vi "Vision Processing.vi"(4 "error in (no error)":errorcluster) -> ()   [LabVIEW 2015]
doc: "This VI runs in parallel to other tasks. It gets images from the camera, processes them for color or shape and use that information to affect robot behavior."
uses:
  <vilib>/Rock Robotics/SystemInterfaces/NetworkCommunication/NetComm_UsageReport_ResourceType.ctl
  <vilib>/Rock Robotics/WPI/Camera/WPI_CameraExposure Values.ctl
  <vilib>/Rock Robotics/WPI/Utilities/WPI_GetSetVariantRefNum.vi
  <vilib>/Rock Robotics/Network Tables/NT Write Boolean.vi
  Robot Global Data.vi
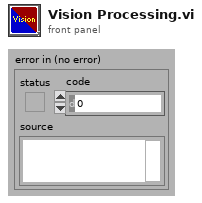
[diagram p1: front panel]
types:
  T1 = typedef "WPI_CameraExposure Values.ctl" = enum16{"Auto", "Flicker-free 50 Hz", "Flicker-free 60 Hz", "Hold current", "Custom"}
  T2 = cluster{"fps":i32, "compression":i32, "compression 2":i32}
  T3 = typedef "NetComm_UsageReport_ResourceType.ctl" = enum8{"Controller", "Module", "Language", "CANPlugin", "Accelerometer", "ADXL345", "AnalogChannel", "AnalogTrigger", "AnalogTriggerOutput", "CANJaguar", "Compressor", "Counter", "Dashboard", "DigitalInput", "DigitalOutput", "DriverStationCIO", "DriverStationEIO", "DriverStationLCD", "Encoder", "GearTooth", "Gyro", "I2C", "Framework", "Jaguar", "Joystick", "Kinect", "KinectStick", "PIDController", "Preferences", "PWM", "Relay", "RobotDrive", "SerialPort", "Servo", "Solenoid", "SPI", "Task", "Ultrasonic", "Victor", "Button", "Command", "AxisCamera", "PCVideoServer", "SmartDashboard", "Talon", "HiTechnicColorSensor", "HiTechnicAccel", "HiTechnicCompass", "SRF08", "AnalogOutput", "Victor SP", "Talon SRX", "CAN Talon SRX", "ADXL362 Accel", "ADXRS450 Gyro", "Rev SPARK", "Mindsensors SD540", "Digital Filter"}
  T4 = enum16{"Update Mode", "Get Image", "Get Image Data"}
  T5 = typedef "WPI_JoystickDevRef.ctl" = cluster{"Device":T6}
  T6 = typedef "WPI_JoystickDeviceEnum.ctl" = enum16{"USB 0", "USB 1", "USB 2", "USB 3", "USB 4", "USB 5"}
  T7 = typedef "WPI_CameraDevRef.ctl" = cluster{"Camera Address":string, "CameraStatus":errorcluster}
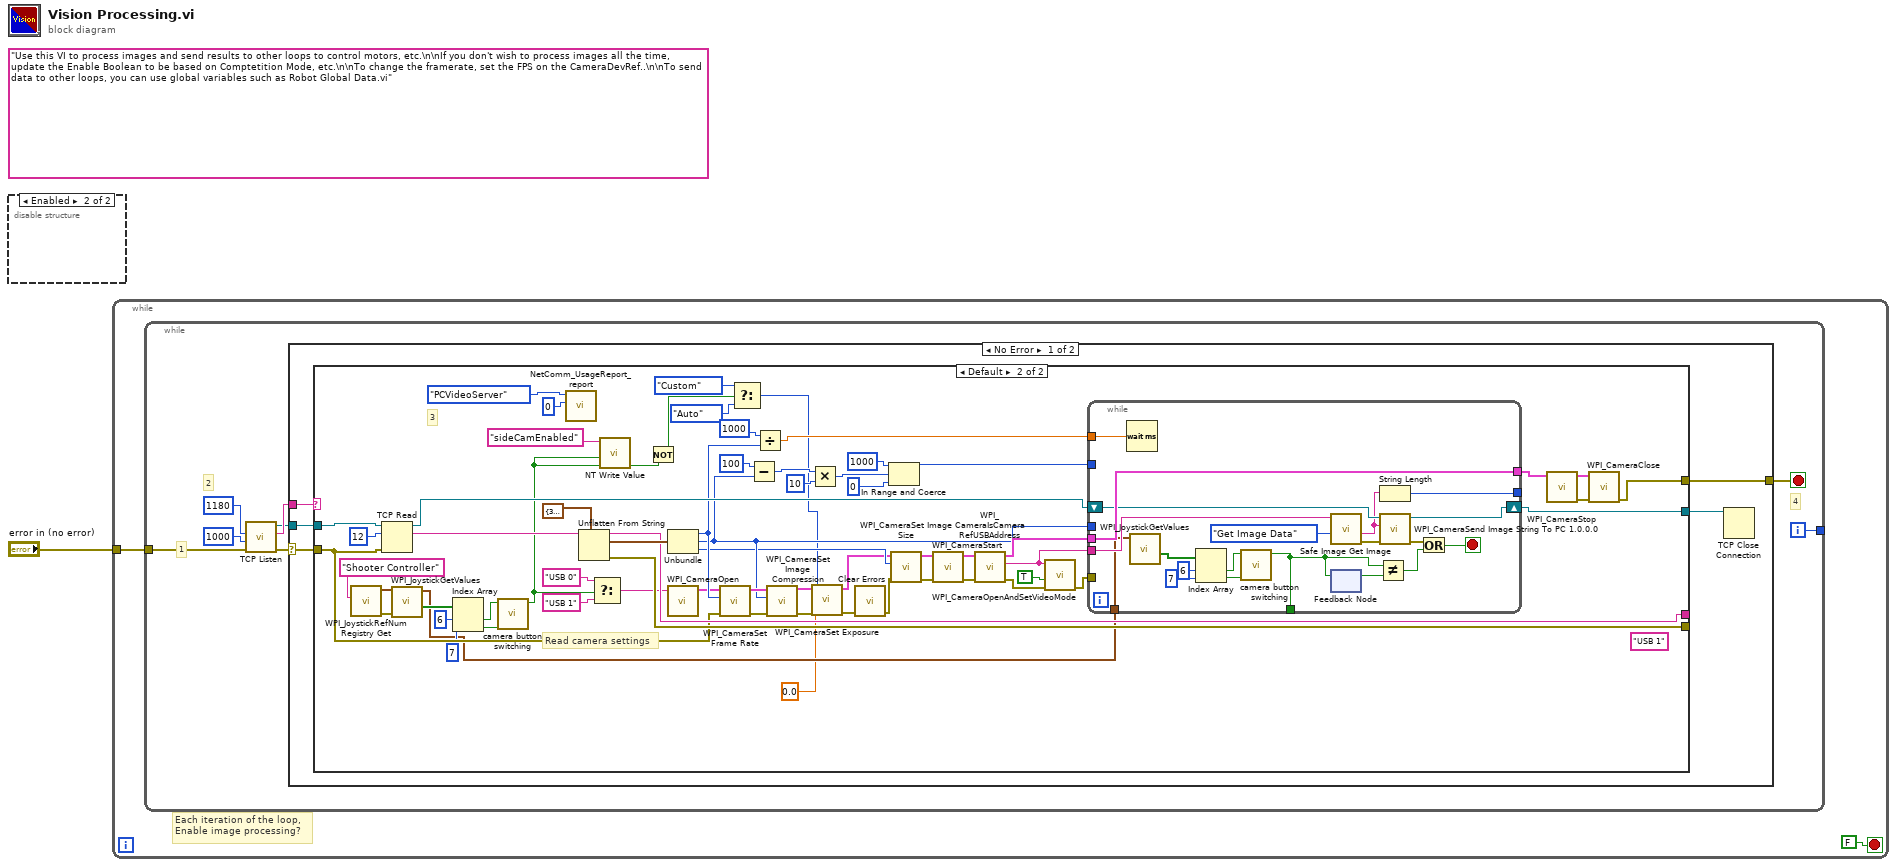
[diagram p0: block diagram]
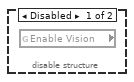
[diagram p2: hidden frame]
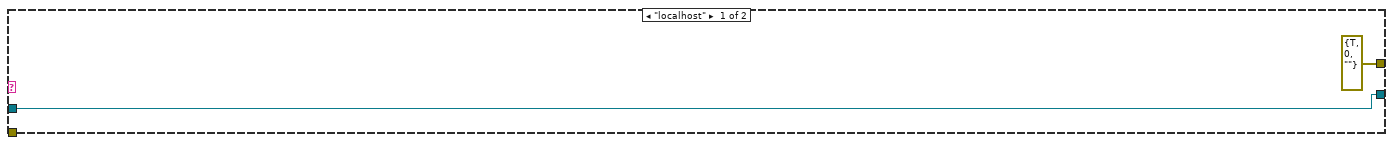
[diagram p3: hidden frame]
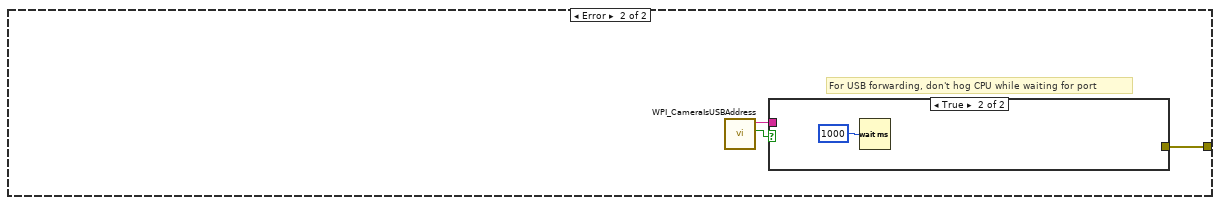
[diagram p4: hidden frame]
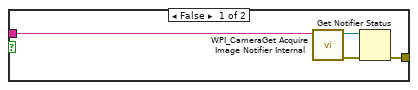
[diagram p5: hidden frame]
diagram:
  (unwired) "Use this VI to process images and send results to other loops to control motors, etc.\n\nIf you don't wish to process images all the time, update the Enable Boolean to be based on Comptetition Mode, etc.\n\nTo change the framerate, set the FPS on the CameraDevRef..\n\nTo send data to other loops, you can use global variables such as Robot Global Data.vi"
  n1 = disable-structure shown="Enabled" {
    frame Disabled {
      n2 = global read "Robot Global Data.vi" "Enable Vision"() -> ()  [unwired: 1 out]
    }
    frame Enabled {
    }
  }
  n3 = while {
    tunnel: "error in (no error)" -> [w2]
    stop <- FALSE stop-if-true
    # "Each iteration of the loop,\nEnable image processing?"
    n4 = while {
      tunnel: w2 -> [w10]
      tunnel: [w4] -> _
      i -> [w4]
      stop <- w8 stop-if-true
      # "4"
      # "1"
      # "2"
      n5 = call <vilib>:"TCP Listen.vi"("error in (no error)"=w10, "timeout ms (wait forever: -1)"=u16 1000 ("port"), "port"=u16 1180) -> ("error out"=w6:errorcluster, "remote address"=w11:string, "connection ID"=w9:refnum<k5>)  [unwired: 1 in, 5 out]
      n6 = case shown="No Error" w6 {
        selector: w6 -> [w12 _]
        tunnel: w11 -> [w16 _]
        tunnel: w9 -> [w15 _]
        tunnel: [w14 w105] -> w8
        frame No Error {
          n7 = case shown="Default" w16 {
            tunnel: w12 -> [_ w51]
            tunnel: w15 -> [w17 w73]
            tunnel: [errorcluster {"status"=TRUE, "code"=0, "source"=""} ("error out 2") w39] -> w14
            tunnel: [w17 w82] -> w13
            tunnel: [_ w53] -> _
            tunnel: [_ w52] -> _
            frame "localhost" {
            }
            frame Default {
              (unwired) "USB 1" ("format string")
              # "Read camera settings"
              # "3"
              n8 = call <vilib>:"WPI_JoystickRefNum Registry Get.vi"("refnum name"="Shooter Controller") -> ("error out"=w37:errorcluster, "JoystickDevRef"=w38:T5)  [unwired: 9 in]
              n9 = TCP Read(connection ID=w73, bytes to read=12, error in (no error)=w51) -> (connection ID out=w72:refnum<k5>, data out=w70:string)  [unwired: 2 in, 1 out]
              n10 = call <vilib>:"WPI_JoystickGetValues.vi"("error in (no error)"=w37, "JoystickDevRef"=w38) -> ("Buttons"=w35:bool[], "JoystickDevRef"=w30:T5)  [unwired: 5 in, 3 out]
              n11 = Index Array(array=w35, index #1=6 ("index"), index #2=7 ("index")) -> (element #1=w31:bool, element #2=w32:bool)
              n12 = call "camera button switching.vi"("Cam 2 Button"=w32, "Cam 1 Button"=w31) -> ("Use Cam 2?"=w23:bool)  [unwired: 9 in]
              n13 = call <vilib>:"NetComm_UsageReport_report.vi"("Instance Number"=u8 0, "Resource Type"=NetComm_UsageReport_ResourceType."PCVideoServer") -> ()  [unwired: 10 in]
              n14 = Unflatten From String(type=T2 {"fps"=30, "compression"=32, "compression 2"=32} ("Camera Settings"), binary string=w70) -> (rest of the binary string=w52:string, value=w65:T2, error out=w53:errorcluster)  [unwired: 3 in]
              n15 = Select(t="USB 0" ("format string"), s=w23, f="USB 1" ("format string")) -> (s? t:f=w41:string)
              n16 = call-poly <vilib>:"NT Write Value.vi"("Boolean"=w23, "Name"="sideCamEnabled") -> ()  [unwired: 9 in, 1 out]
              n17 = Not(x=w23) -> (.not. x?=w19:bool)
              n18 = Unbundle(w65) -> ("fps"=w50:i32, "compression"=w49:i32, "compression 2"=w48:i32)
              n19 = call <vilib>:"WPI_CameraOpen.vi"("Camera Address"=w41) -> ("CameraDevRef"=w40:T7)  [unwired: 1 in, 9 out]
              n20 = call <vilib>:"WPI_CameraSet Frame Rate.vi"("error in (no error)"=w51, "Frame Rate (fps)"=w50, "CameraDevRef"=w40) -> ("error out"=w67:errorcluster, "CameraDevRef Out"=w69:T7)  [unwired: 7 in]
              n21 = Select(t=WPI_CameraExposure_Values."Custom" ("Exposure"), s=w19, f=WPI_CameraExposure_Values."Auto") -> (s? t:f=w25:T1)
              n22 = Subtract(x=100, y=w49) -> (x-y=w58:i32)
              n23 = Divide(x=u16 1000 ("port"), y=w50) -> (x/y=w63:dbl)
              n24 = call <vilib>:"WPI_CameraSet Image Compression.vi"("error in (no error)"=w67, "Compression"=w49, "CameraDevRef"=w69) -> ("error out"=w21:errorcluster, "CameraDevRef Out"=w22:T7)  [unwired: 7 in]
              n25 = Multiply(x=w58, y=10) -> (x*y=w60:i32)
              n26 = call <vilib>:"WPI_CameraSet Exposure.vi"("error in (no error)"=w21, "Exposure (%)"=0.0, "Exposure"=w25, "CameraDevRef"=w22) -> ("error out"=w28:errorcluster, "CameraDevRef Out"=w29:T7)  [unwired: 6 in]
              n27 = call <vilib>:"Clear Errors.vi"("error in (no error)"=w28) -> ("error out"=w54:errorcluster)  [unwired: 5 in, 1 out]
              n28 = In Range and Coerce(upper limit=1000, x=w60, lower limit=0) -> (coerced(x)=w56:i32)  [unwired: 1 out]
              n29 = call <vilib>:"WPI_CameraSet Image Size.vi"("error in (no error)"=w54, "Image Size"=w48, "CameraDevRef"=w29) -> ("error out"=w66:errorcluster, "CameraDevRef Out"=w68:T7)  [unwired: 7 in]
              n30 = call <vilib>:"WPI_CameraStart.vi"("error in (no error)"=w66, "CameraDevRef"=w68) -> ("error out"=w77:errorcluster, "CameraDevRef"=w75:T7)  [unwired: 8 out]
              n31 = call <vilib>:"WPI_CameraIsCameraRefUSBAddress.vi"("error in (no error)"=w77, "CameraDevRef"=w75) -> ("error out"=w76:errorcluster, "Camera Address Out"=w78:string, "CameraDevRef out"=w74:T7)  [unwired: 6 in, 1 out]
              n32 = call <vilib>:"WPI_CameraOpenAndSetVideoMode.vi"("error in (no error)"=w76, "USB JPEG"=TRUE, "Camera Address Out"=w78) -> ("error out"=w47:errorcluster)  [unwired: 8 in]
              n33 = while {
                tunnel: w78 -> [w90]
                shift-right: [w102] -> w82
                shift-left: w72 -> [w99]
                tunnel: [w101] -> w81
                tunnel: w74 -> [w101]
                tunnel: w56 -> [_]
                tunnel: w63 -> [w100]
                tunnel: [w98] -> _
                tunnel: w49 -> [_]
                tunnel: w47 -> [_]
                tunnel: [w87] -> _
                tunnel: w30 -> [w85]
                stop <- w91 stop-if-true
                n34 = Wait (ms)(milliseconds to wait=w100) -> ()  [unwired: 1 out]
                n35 = call <vilib>:"WPI_JoystickGetValues.vi"("JoystickDevRef"=w85) -> ("Buttons"=w86:bool[])  [unwired: 6 in, 4 out]
                n36 = Index Array(array=w86, index #1=6 ("index"), index #2=7 ("index")) -> (element #1=w84:bool, element #2=w83:bool)
                n37 = call "camera button switching.vi"("Cam 2 Button"=w83, "Cam 1 Button"=w84) -> ("Use Cam 2?"=w87:bool)  [unwired: 9 in]
                n38 = call <vilib>:"Safe Image Get Image.vi"("Operation"=T4."Get Image Data", "Session In"=w90) -> ("error out"=w95:errorcluster, "Image Data String"=w96:string)  [unwired: 6 in, 2 out]
                n39 = feedback-in #1(w87) -> ()
                n40 = feedback #1() -> (w94:bool)  [unwired: 1 in]
                n41 = Not Equal?(x=w87, y=w94) -> (x != y?=w93:bool)
                n42 = String Length(string=w96) -> (length=w98:i32)
                n43 = call <vilib>:"WPI_CameraSend Image String To PC 1.0.0.0.vi"("error in (no error)"=w95, "String"=w96, "TCP Connection ID"=w99) -> ("error out"=w92:errorcluster, "TCP Connection ID out"=w102:refnum<k5>)  [unwired: 7 out]
                n44 = Or(x=w92, y=w93) -> (x .or. y?=w91:bool)
              }
              n45 = call <vilib>:"WPI_CameraStop.vi"("CameraDevRef"=w81) -> ("error out"=w44:errorcluster, "CameraDevRef"=w45:T7)  [unwired: 1 in, 8 out]
              n46 = call <vilib>:"WPI_CameraClose.vi"("error in (no error)"=w44, "CameraDevRef"=w45) -> ("error out"=w39:errorcluster)  [unwired: 9 in]
            }
          }
          n47 = TCP Close Connection(connection ID=w13) -> ()  [unwired: 1 in, 3 out]
        }
        frame Error {
          # "For USB forwarding, don't hog CPU while waiting for port"
          n48 = call <vilib>:"WPI_CameraIsUSBAddress.vi"() -> ("USB?"=w103:bool, "Camera Address Out"=w104:string)  [unwired: 9 in, 1 out]
          n49 = case shown="True" w103 {
            tunnel: [w109 _] -> w105
            tunnel: w104 -> [w106 _]
            frame False {
              n50 = call <vilib>:"WPI_CameraGet Acquire Image Notifier Internal.vi"("Camera Address"=w106) -> ("error out"=w107:errorcluster, "Acquire Image Notifier"=w108:refnum<notifier>)  [unwired: 1 in, 8 out]
              n51 = Get Notifier Status(notifier=w108, error in (no error)=w107) -> (error out=w109:errorcluster)  [unwired: 4 out]
            }
            frame True {
              n52 = Wait (ms)(milliseconds to wait=u32 1000) -> ()  [unwired: 1 out]
            }
          }
        }
      }
    }
  }
